vi "Send User Event-Panel Resize.vi"(7 "Message Priority (Normal)":T5=enum."Normal", 8 "error in (no error)":errorcluster, 10 "Panel Resize Data":T1={"OldBnds"={"Left"=0, "Top"=0, "Right"=0, "Bottom"=0}, "NewBnds"={"Left"=0, "Top"=0, "Right"=0, "Bottom"=0}, "Act"=enum."Resized", "PrevState"=enum."Standard"}, 11 "Message Enqueuer":refnum<class "Message Enqueuer.lvclass">) -> (0 "error out":errorcluster, 3 "Message Enqueuer out":refnum<class "Message Enqueuer.lvclass">)   [LabVIEW 2021, in "Appearance Actor.lvlib" / "User Event-Panel Resize Msg.lvclass"]
doc: "This VI sends the message to an actor."
uses:
  User Event-Panel Resize Msg.lvclass
  <vilib>/ActorFramework/Message Enqueuer/Message Enqueuer.lvclass
  <vilib>/ActorFramework/Message Enqueuer/Message Priority.ctl
  Appearance Actor/Typedefs/User Event-Panel Resize-Data--cluster.ctl
  <vilib>/Utility/miscctls.llb/LVRectTypeDef.ctl
  <vilib>/event_ctls.llb/sizeaction.ctl
  <vilib>/event_ctls.llb/panelstate.ctl
  C:/Program Files (x86)/National Instruments/LabVIEW 2021/vi.lib/ActorFramework/Message/Message.lvclass
  User Event-Panel Resize Msg.lvclass/User Event-Panel Resize Msg.ctl
  <vilib>/ActorFramework/Message Enqueuer/Message Enqueuer.lvclass/Message Enqueuer.ctl
  <vilib>/ActorFramework/Message Priority Queue/Priority Enqueue.vi
  Appearance Actor/Appearance Actor.lvclass
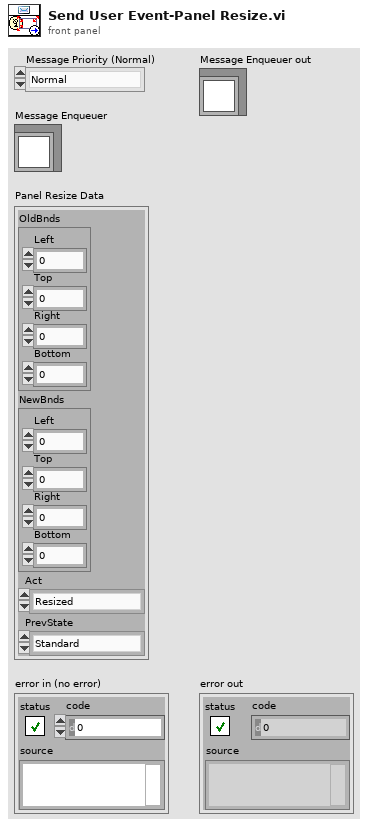
[diagram p1: front panel]
types:
  T1 = typedef "Appearance Actor.lvlib/Appearance Actor.lvclass/User Event-Panel Resize-Data--cluster.ctl" = cluster{"OldBnds":T2, "NewBnds":T2, "Act":T3, "PrevState":T4}
  T2 = typedef "LVRectTypeDef.ctl" = cluster{"Left":i16, "Top":i16, "Right":i16, "Bottom":i16}
  T3 = typedef "sizeaction.ctl" = enum32{"Minimized", "Maximized", "Resized"}
  T4 = typedef "panelstate.ctl" = enum32{"Standard", "Minimized", "Maximized"}
  T5 = typedef "Actor Framework.lvlib/Message Enqueuer.lvclass/Message Priority.ctl" = enum16{"Low", "Normal", "High"}
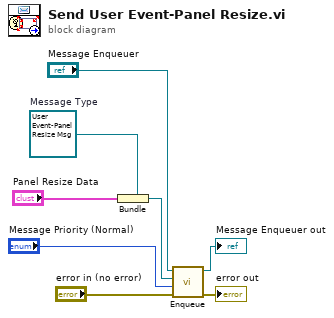
[diagram p0: block diagram]
diagram:
  w2 = refnum<class "User Event-Panel Resize Msg.lvclass"> refnum  # Message Type
  n1 = Bundle(cluster=w2, "Panel Resize Data") -> (w3:refnum<class "User Event-Panel Resize Msg.lvclass">)
  n2 = call <vilib>:"Enqueue.vi"("error in (no error)"="error in (no error)", "Message Priority (Normal)"="Message Priority (Normal)", "Message"=w3, "Message Enqueuer in"="Message Enqueuer") -> ("error out"=→"error out":errorcluster, "Message Enqueuer out"=→"Message Enqueuer out":refnum<class "Message Enqueuer.lvclass">)  [unwired: 6 in]
